vi "Msg.vi"(7 "jettl in":refnum<class "jettl.lvclass">, 11 "Msg Strategy in":refnum<class "Msg Strategy.lvclass">) -> (5 "jettl out":refnum<class "jettl.lvclass">)   [LabVIEW 2021, in "jettl.lvlib" / "Msg Strategy.lvclass"]
uses:
  Msg Strategy.lvclass
  jettl/jettl.lvclass
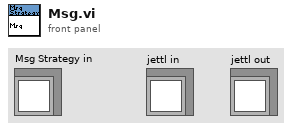
[diagram p1: front panel]
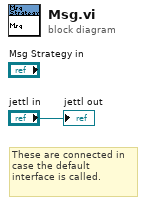
[diagram p0: block diagram]
diagram:
  # "These are connected in case the default interface is called."
  "jettl out" <- "jettl in"
